vi "module timing suffix set.vi"(9 "mod alias":string, 10 "mod id":string, 11 "eng id":string) -> (3 "names":string[](array[string]))   [LabVIEW 2013, in "Standard Engine Configuration.lvclass"]
uses:
  Standard Engine Configuration.lvclass
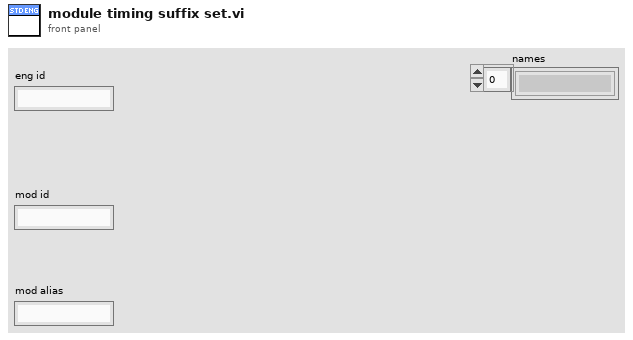
[diagram p1: front panel]
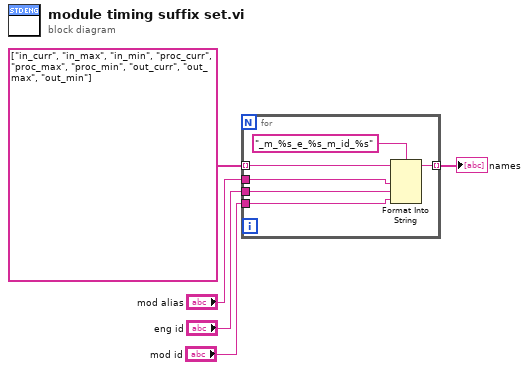
[diagram p0: block diagram]
diagram:
  n1 = for {
    tunnel: [w11] -> w5 mode=indexing
    tunnel: string[] ["in_curr", "in_max", "in_min", "proc_curr", "proc_max", "proc_min", "out_curr", "out_max", "out_min"] -> [w9] mode=indexing
    tunnel: "mod alias" -> [w10]
    tunnel: "eng id" -> [w8]
    tunnel: "mod id" -> [w7]
    n2 = Format Into String(format string="_m_%s_e_%s_m_id_%s", initial string=w9, w10, w8, w7) -> (resulting string=w11:string)  [unwired: 1 in, 1 out]
  }
  "names" <- w5
